vi "Export dat - tag.vi"(8 "Error In":errorcluster, 9 "Workspace":path, 10 "Index":T1 {"IV"."IV properties"."Settling" min=0.0 max=65535.0; "CV"."CV properties"."V range" items=["10mV"=0.01, "100mV"=0.1, "1V"=1.0, "10V"=10.0]; "CV"."CV properties"."I range" items=["100nA"=-7.0, "1µA"=-6.0, "10µA"=-5.0, "100µA"=-4.0, "1mA"=-3.0, "10mA"=-2.0]; "LDLTS"."LDLTS properties"."V range" items=["10mV"=0.01, "100mV"=0.1, "1V"=1.0, "10V"=10.0]; "LDLTS"."LDLTS properties"."I range" items=["100nA"=-7.0, "1µA"=-6.0, "10µA"=-5.0, "100µA"=-4.0, "1mA"=-3.0, "10mA"=-2.0]; "Conv DLTS"."DLTS properties"."V range" items=["10mV"=0.01, "100mV"=0.1, "1V"=1.0, "10V"=10.0]; "Conv DLTS"."DLTS properties"."I range" items=["10mV"=0.01, "100mV"=0.1, "1V"=1.0, "10V"=10.0]}, 11 "Measurement tag":string) -> (0 "Error Out":errorcluster)   [LabVIEW 2019]
doc: "Handles export of measurement (identified by a tag) to a .dat file, displays a GUI window"
uses:
  Type defs/Session internal index Type Def.ctl
  Type defs/IV measurement Type Def.ctl
  Type defs/IV properties Type Def.ctl
  Type defs/CV measurement Type Def.ctl
  Type defs/CV properties Type Def.ctl
  Type defs/LDLTS measurement Type Def.ctl
  Type defs/LDLTS properties Type Def.ctl
  Type defs/cDLTS measurement Type Def.ctl
  Type defs/DLTS properties Type Def.ctl
  <vilib>/Utility/sysdir.llb/System Directory Type.ctl
  <vilib>/Utility/file.llb/Write Delimited Spreadsheet (string).vi
  <vilib>/Utility/file.llb/Write Delimited Spreadsheet (DBL).vi
panel:
  out "String":string
  in  "Path":path caption="Export file as:"
  in  "Export":bool
  in  "Cancel":bool
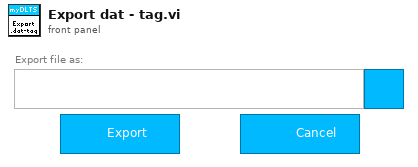
[diagram p1: front panel]
types:
  T1 = typedef "Session internal index Type Def.ctl" = cluster{"IV":T2[], "CV":T4[], "LDLTS":T6[], "Conv DLTS":T8[]}
  T2 = typedef "IV measurement Type Def.ctl" = cluster{"Name":string, "Comment":string, "Time":timestamp, "Folder":path, "IV properties":T3, "GUID":string}
  T3 = typedef "IV properties Type Def.ctl" = cluster{"T":dbl[unit], "Vstart":dbl[unit], "Vstop":dbl[unit], "Vpoints":dbl, "Settling":dbl[unit], "I limit":dbl[unit], "Log mapping":bool, "Averaging":dbl}
  T4 = typedef "CV measurement Type Def.ctl" = cluster{"Name":string, "Comment":string, "Time":timestamp, "Folder":path, "CV properties":T5, "GUID":string}
  T5 = typedef "CV properties Type Def.ctl" = cluster{"T":dbl[unit], "Vstart":dbl[unit], "Vstop":dbl[unit], "Vpoints":dbl, "Precision":enum16{"Low (Fast)", "Normal", "High (Slow)"}, "Test signal":dbl[unit], "Auto I range":bool, "Test frequency":dbl[unit], "I range":dbl, "V range":dbl[unit], "Log mapping":bool, "Rel perm":dbl, "Area":dbl[unit]}
  T6 = typedef "LDLTS measurement Type Def.ctl" = cluster{"Name":string, "Comment":string, "Time":timestamp, "Folder":path, "LDLTS properties":T7, "GUID":string}
  T7 = typedef "LDLTS properties Type Def.ctl" = cluster{"T":dbl[unit], "Test signal":dbl[unit], "Test frequency":dbl[unit], "Bandwidth":dbl[unit], "Averaging":dbl, "Vbias":dbl[unit], "Vpulse":dbl[unit], "pulse length":dbl[unit], "Pulse 2":bool, "Vpulse 2":dbl[unit], "pulse length 2":dbl[unit], "I range":dbl, "V range":dbl[unit], "Sampling rate":dbl[unit], "Acq. delay":dbl[unit], "Sampling time":dbl[unit]}
  T8 = typedef "cDLTS measurement Type Def.ctl" = cluster{"Name":string, "Comment":string, "Time":timestamp, "Folder":path, "DLTS properties":T9, "GUID":string}
  T9 = typedef "DLTS properties Type Def.ctl" = cluster{"Tstart":dbl[unit], "Instant start":bool, "Tstop":dbl[unit], "T rate":dbl[unit], "Test signal":dbl[unit], "Test frequency":dbl[unit], "Bandwidth":dbl[unit], "Averaging":dbl, "Vbias":dbl[unit], "Vpulse":dbl[unit], "pulse length":dbl[unit], "Pulse 2":bool, "Vpulse 2":dbl[unit], "pulse length 2":dbl[unit], "I range":dbl, "V range":dbl[unit], "Emission rate":dbl[unit][], "Sampling rate":dbl[unit], "Acq. delay":dbl[unit]}
  T10 = enum32{"existing file", "new file", "new or existing file", "existing dir", "new dir", "new or existing dir", "existing file (use LLBs)", "new file (use LLBs)", "new or existing file (use LLBs)", "new or existing file or directory (use LLBs)", "existing dir (use LLBs)", "new dir (use LLBs)", "new or existing dir (use LLBs)", "existing file or dir", "new file or dir", "new or existing file or dir", "existing file or dir (use LLBs)", "new file or dir (use LLBs)"}
  T11 = typedef "System Directory Type.ctl" = i32
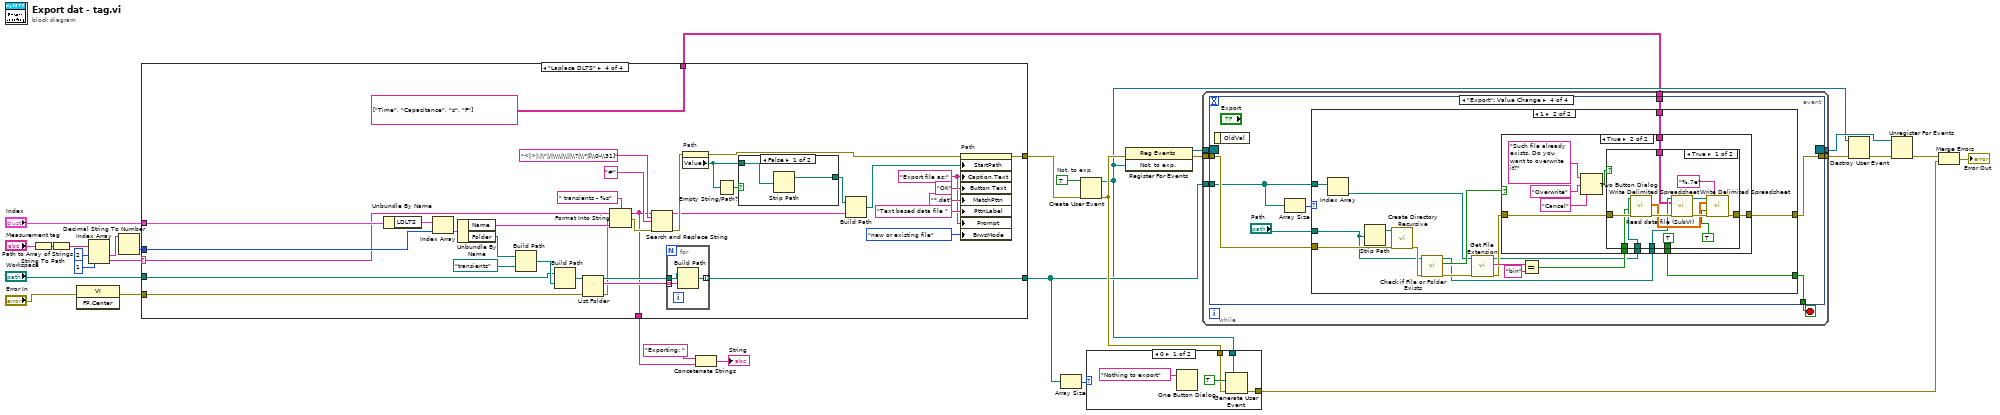
[diagram p0: block diagram]
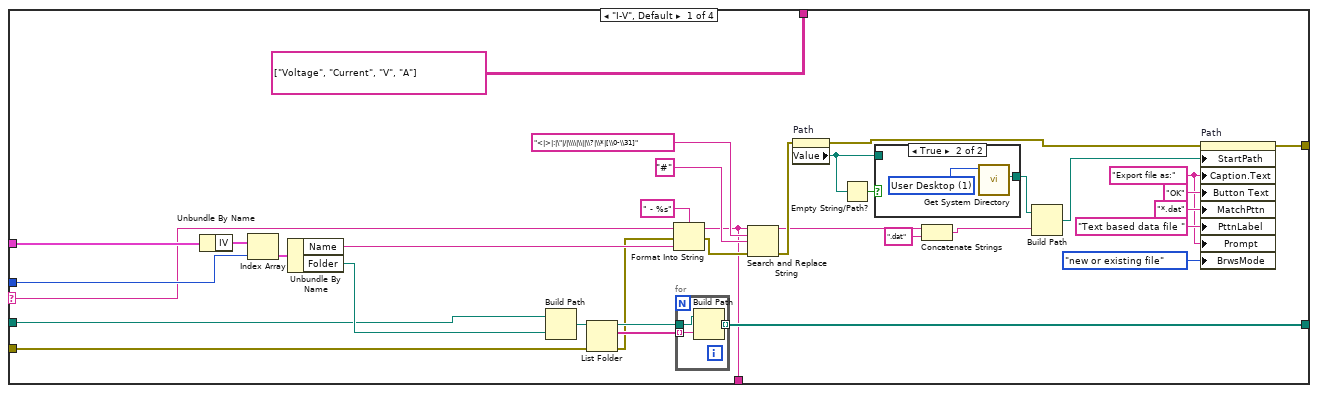
[diagram p3: hidden frame]
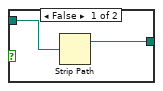
[diagram p4: hidden frame]
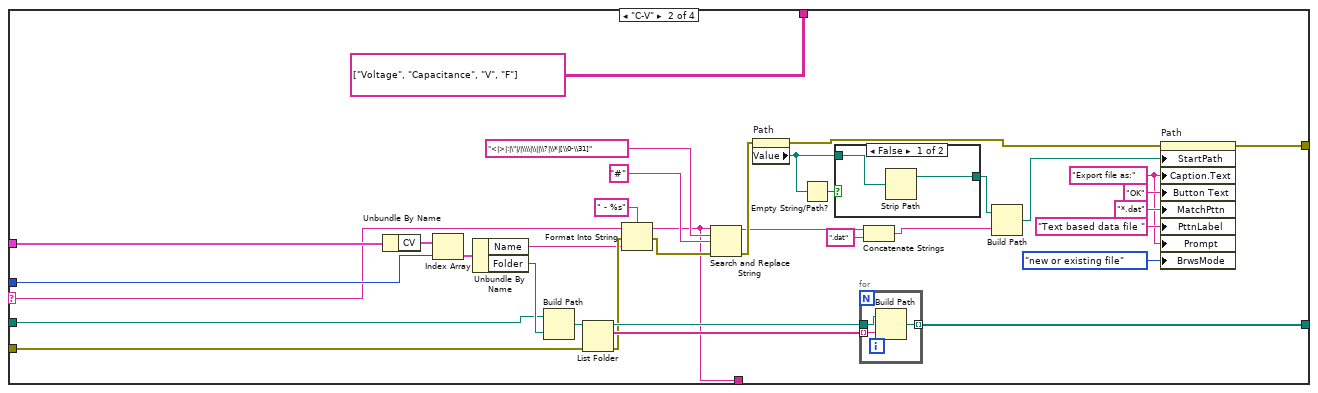
[diagram p5: hidden frame]
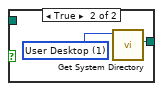
[diagram p6: hidden frame]
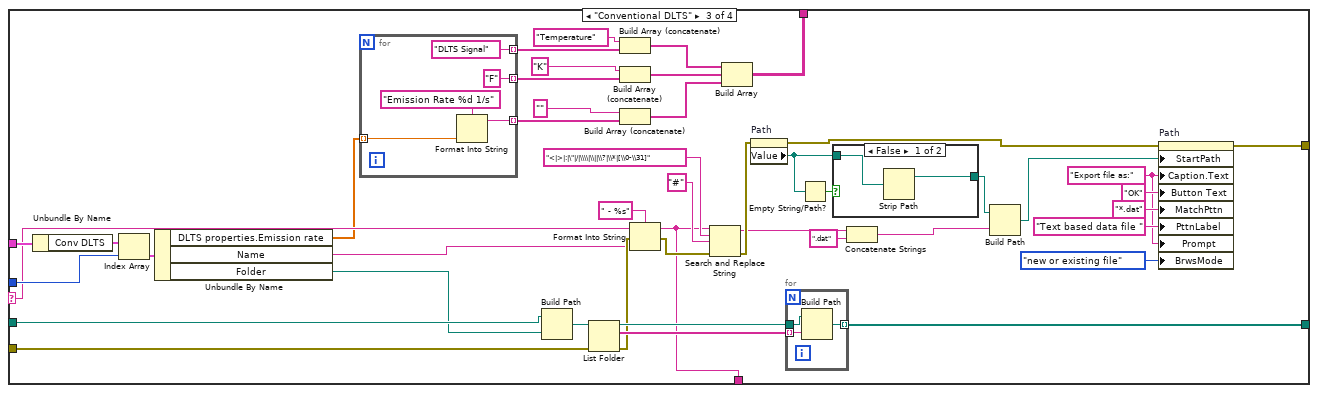
[diagram p7: hidden frame]
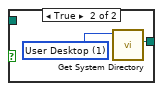
[diagram p8: hidden frame]
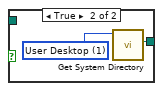
[diagram p9: hidden frame]
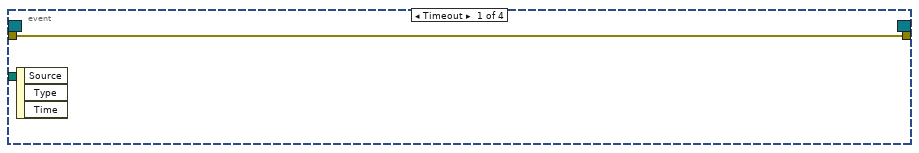
[diagram p10: hidden frame]
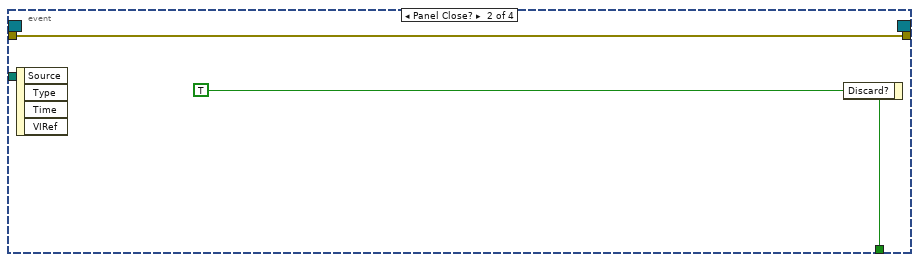
[diagram p11: hidden frame]
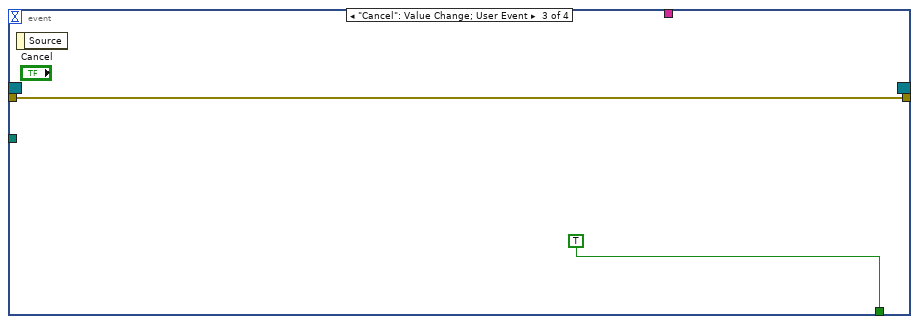
[diagram p12: hidden frame]
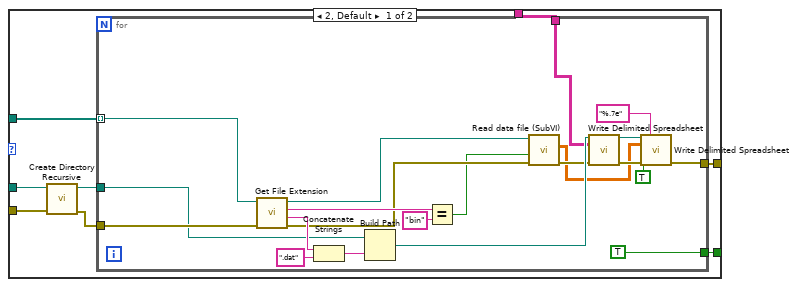
[diagram p13: hidden frame]
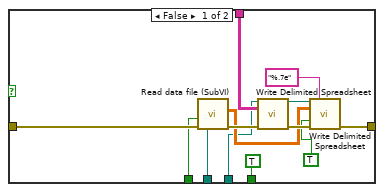
[diagram p14: hidden frame]
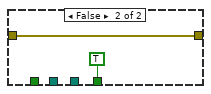
[diagram p15: hidden frame]
diagram:
  w19 = TRUE  # Not. to exp.
  n1 = String To Path(string="Measurement tag") -> (path=w30:path)
  n2 = Path to Array of Strings(0:w30) -> (2:w29:string[])  [unwired: 1 out]
  n3 = invoke class="VI" method="FP.Center"(error in="Error In") -> (error out=w2:errorcluster)  [unwired: 2 in, 2 out]
  n4 = Index Array(array=w29, index #1=2 ("index"), index #2=1 ("index")) -> (element #1=w24:string, element #2=w25:string)
  n5 = Decimal String To Number(string=w24) -> (number=w22:i32)  [unwired: 2 in, 1 out]
  n6 = case shown="\"Laplace DLTS\"" w25 {
    selector: w25 -> [w59 w101 w153 w200]
    tunnel: "Index" -> [w65 w107 w159 w206]
    tunnel: w22 -> [w63 w105 w157 w204]
    tunnel: [w51 w93 w146 w193] -> w14
    tunnel: w2 -> [w49 w91 w144 w191]
    tunnel: [w48 w90 w143 w190] -> w16
    tunnel: "Workspace" -> [w40 w82 w135 w180]
    tunnel: [w36 w75 w131 w173] -> w6
    tunnel: [string[][] [["Voltage", "Current"], ["V", "A"]] string[][] [["Voltage", "Capacitance"], ["V", "F"]] w115 string[][] [["Time", "Capacitance"], ["s", "F"]]] -> w1
    frame "I-V", Default {
      w44 = "Export file as:"
      n7 = Unbundle By Name(w65) -> ("IV"=w64:T2[])
      n8 = Index Array(array=w64, index=w63) -> (element=w62:T2)
      n9 = Unbundle By Name(w62) -> ("Name"=w38:string, "Folder"=w52:path)
      n10 = Build Path(base path=w40, name or relative path=w52) -> (appended path=w42:path)
      n11 = List Folder(path=w42, error in=w49) -> (path out=w41:path, filenames=w50:string[], error out=w32:errorcluster)  [unwired: 2 in, 1 out]
      n12 = Format Into String(format string=" - %s", initial string=w59, error in=w32, w38) -> (resulting string=w36:string, error out=w37:errorcluster)
      n13 = for {
        tunnel: w41 -> [w68]
        tunnel: [w67] -> w51 mode=indexing
        tunnel: w50 -> [w66] mode=indexing
        n14 = Build Path(base path=w68, name or relative path=w66) -> (appended path=w67:path)
      }
      n15 = Search and Replace String(input string=w36, search string="<|>|:|\"|/|\\\\|\\||\\?|\\*|[\\0-\\31]", replace string="#" ("replace string (\"\")"), error in=w37) -> (result string=w35:string, error out=w39:errorcluster)  [unwired: 4 in, 2 out]
      n16 = property on="Path" class="Path"(error in=w39) -> (error out=w53:errorcluster, "Value"=w60:path)  [unwired: 1 in, 1 out]
      n17 = Empty String/Path?(string/path=w60) -> (empty?=w61:bool)
      n18 = case shown="True" w61 {
        tunnel: w60 -> [w70 _]
        tunnel: [w69 w71] -> w55
        frame False {
          n19 = Strip Path(path=w70) -> (stripped path=w69:path)  [unwired: 1 out]
        }
        frame True {
          w72 = T11 1 items=["User Home"=0, "User Desktop"=1, "User Documents"=2, "User Application Data"=3, "User Preferences"=4, "User Temporary"=5, "Public Documents"=6, "Public Application Data"=7, "Public Preferences"=8, "Public Cache"=13, "System Core Libraries"=9, "System Installed Libraries"=10, "Application Files"=11, "Boot Volume Root"=12] ("system directory type")
          n20 = call <vilib>:"Get System Directory.vi"("system directory type"=w72) -> ("system directory"=w71:path)  [unwired: 10 in]
        }
      }
      n21 = Concatenate Strings(w35, ".dat" ("string")) -> (w34:string)
      n22 = Build Path(base path=w55, name or relative path=w34) -> (appended path=w54:path)
      n23 = property on="Path" class="Path"(error in=w53, "StartPath"=w54, "Caption.Text"=w44, "Button Text"="OK", "MatchPttn"="*.dat", "PttnLabel"="Text based data file ", "Prompt"=w44, "BrwsMode"=T10."new or existing file" ("Browse Options:Selection Mode")) -> (error out=w48:errorcluster)  [unwired: 1 in, 1 out]
    }
    frame "C-V" {
      w86 = "Export file as:"
      n24 = Unbundle By Name(w107) -> ("CV"=w106:T4[])
      n25 = Index Array(array=w106, index=w105) -> (element=w104:T4)
      n26 = Unbundle By Name(w104) -> ("Name"=w76:string, "Folder"=w94:path)
      n27 = Build Path(base path=w82, name or relative path=w94) -> (appended path=w84:path)
      n28 = List Folder(path=w84, error in=w91) -> (path out=w83:path, filenames=w92:string[], error out=w78:errorcluster)  [unwired: 2 in, 1 out]
      n29 = Format Into String(format string=" - %s", initial string=w101, error in=w78, w76) -> (resulting string=w75:string, error out=w77:errorcluster)
      n30 = Search and Replace String(input string=w75, search string="<|>|:|\"|/|\\\\|\\||\\?|\\*|[\\0-\\31]", replace string="#" ("replace string (\"\")"), error in=w77) -> (result string=w74:string, error out=w79:errorcluster)  [unwired: 4 in, 2 out]
      n31 = property on="Path" class="Path"(error in=w79) -> (error out=w95:errorcluster, "Value"=w102:path)  [unwired: 1 in, 1 out]
      n32 = Empty String/Path?(string/path=w102) -> (empty?=w103:bool)
      n33 = case shown="False" w103 {
        tunnel: w102 -> [w112 _]
        tunnel: [w111 w113] -> w97
        frame False {
          n34 = Strip Path(path=w112) -> (stripped path=w111:path)  [unwired: 1 out]
        }
        frame True {
          w114 = T11 1 items=["User Home"=0, "User Desktop"=1, "User Documents"=2, "User Application Data"=3, "User Preferences"=4, "User Temporary"=5, "Public Documents"=6, "Public Application Data"=7, "Public Preferences"=8, "Public Cache"=13, "System Core Libraries"=9, "System Installed Libraries"=10, "Application Files"=11, "Boot Volume Root"=12] ("system directory type")
          n35 = call <vilib>:"Get System Directory.vi"("system directory type"=w114) -> ("system directory"=w113:path)  [unwired: 10 in]
        }
      }
      n36 = for {
        tunnel: w83 -> [w110]
        tunnel: [w109] -> w93 mode=indexing
        tunnel: w92 -> [w108] mode=indexing
        n37 = Build Path(base path=w110, name or relative path=w108) -> (appended path=w109:path)
      }
      n38 = Concatenate Strings(w74, ".dat" ("string")) -> (w80:string)
      n39 = Build Path(base path=w97, name or relative path=w80) -> (appended path=w96:path)
      n40 = property on="Path" class="Path"(error in=w95, "StartPath"=w96, "Caption.Text"=w86, "Button Text"="OK", "MatchPttn"="*.dat", "PttnLabel"="Text based data file ", "Prompt"=w86, "BrwsMode"=T10."new or existing file" ("Browse Options:Selection Mode")) -> (error out=w90:errorcluster)  [unwired: 1 in, 1 out]
    }
    frame "Conventional DLTS" {
      w139 = "Export file as:"
      n41 = Unbundle By Name(w159) -> ("Conv DLTS"=w158:T8[])
      n42 = Index Array(array=w158, index=w157) -> (element=w156:T8)
      n43 = Unbundle By Name(w156) -> ("DLTS properties.Emission rate"=w116:dbl[unit][], "Name"=w127:string, "Folder"=w117:path)
      n44 = for {
        tunnel: w116 -> [w164] mode=indexing
        tunnel: [w162] -> w123 mode=indexing
        tunnel: ["DLTS Signal"] -> w121 mode=indexing
        tunnel: ["F"] -> w122 mode=indexing
        n45 = Format Into String(format string="Emission Rate %d 1/s", w164) -> (resulting string=w162:string)  [unwired: 2 in, 1 out]
      }
      n46 = Build Path(base path=w135, name or relative path=w117) -> (appended path=w136:path)
      n47 = List Folder(path=w136, error in=w144) -> (path out=w137:path, filenames=w145:string[], error out=w134:errorcluster)  [unwired: 2 in, 1 out]
      n48 = Build Array (concatenate)("Temperature", w121) -> (w118:string[])
      n49 = Build Array (concatenate)("K", w122) -> (w119:string[])
      n50 = Build Array (concatenate)("", w123) -> (w120:string[])
      n51 = Format Into String(format string=" - %s", initial string=w153, error in=w134, w127) -> (resulting string=w131:string, error out=w133:errorcluster)
      n52 = Search and Replace String(input string=w131, search string="<|>|:|\"|/|\\\\|\\||\\?|\\*|[\\0-\\31]", replace string="#" ("replace string (\"\")"), error in=w133) -> (result string=w128:string, error out=w132:errorcluster)  [unwired: 4 in, 2 out]
      n53 = Build Array(w118, w119, w120) -> (w115:string[][])
      n54 = property on="Path" class="Path"(error in=w132) -> (error out=w147:errorcluster, "Value"=w154:path)  [unwired: 1 in, 1 out]
      n55 = for {
        tunnel: w137 -> [w167]
        tunnel: [w166] -> w146 mode=indexing
        tunnel: w145 -> [w165] mode=indexing
        n56 = Build Path(base path=w167, name or relative path=w165) -> (appended path=w166:path)
      }
      n57 = Empty String/Path?(string/path=w154) -> (empty?=w155:bool)
      n58 = case shown="False" w155 {
        tunnel: w154 -> [w169 _]
        tunnel: [w168 w170] -> w149
        frame False {
          n59 = Strip Path(path=w169) -> (stripped path=w168:path)  [unwired: 1 out]
        }
        frame True {
          w171 = T11 1 items=["User Home"=0, "User Desktop"=1, "User Documents"=2, "User Application Data"=3, "User Preferences"=4, "User Temporary"=5, "Public Documents"=6, "Public Application Data"=7, "Public Preferences"=8, "Public Cache"=13, "System Core Libraries"=9, "System Installed Libraries"=10, "Application Files"=11, "Boot Volume Root"=12] ("system directory type")
          n60 = call <vilib>:"Get System Directory.vi"("system directory type"=w171) -> ("system directory"=w170:path)  [unwired: 10 in]
        }
      }
      n61 = Concatenate Strings(w128, ".dat" ("string")) -> (w129:string)
      n62 = Build Path(base path=w149, name or relative path=w129) -> (appended path=w148:path)
      n63 = property on="Path" class="Path"(error in=w147, "StartPath"=w148, "Caption.Text"=w139, "Button Text"="OK", "MatchPttn"="*.dat", "PttnLabel"="Text based data file ", "Prompt"=w139, "BrwsMode"=T10."new or existing file" ("Browse Options:Selection Mode")) -> (error out=w143:errorcluster)  [unwired: 1 in, 1 out]
    }
    frame "Laplace DLTS" {
      w186 = "Export file as:"
      n64 = Unbundle By Name(w206) -> ("LDLTS"=w205:T6[])
      n65 = Index Array(array=w205, index=w204) -> (element=w203:T6)
      n66 = Unbundle By Name(w203) -> ("Name"=w178:string, "Folder"=w183:path)
      n67 = Build Path(base path=w183, name or relative path=path "transients") -> (appended path=w181:path)
      n68 = Build Path(base path=w180, name or relative path=w181) -> (appended path=w184:path)
      n69 = List Folder(path=w184, error in=w191) -> (path out=w179:path, filenames=w192:string[], error out=w177:errorcluster)  [unwired: 2 in, 1 out]
      n70 = Format Into String(format string=" transients - %s", initial string=w200, error in=w177, w178) -> (resulting string=w173:string, error out=w176:errorcluster)
      n71 = Search and Replace String(input string=w173, search string="<|>|:|\"|/|\\\\|\\||\\?|\\*|[\\0-\\31]", replace string="#" ("replace string (\"\")"), error in=w176) -> (result string=w174:string, error out=w175:errorcluster)  [unwired: 4 in, 2 out]
      n72 = for {
        tunnel: w179 -> [w209]
        tunnel: [w208] -> w193 mode=indexing
        tunnel: w192 -> [w207] mode=indexing
        n73 = Build Path(base path=w209, name or relative path=w207) -> (appended path=w208:path)
      }
      n74 = property on="Path" class="Path"(error in=w175) -> (error out=w194:errorcluster, "Value"=w201:path)  [unwired: 1 in, 1 out]
      n75 = Empty String/Path?(string/path=w201) -> (empty?=w202:bool)
      n76 = case shown="False" w202 {
        tunnel: w201 -> [w211 _]
        tunnel: [w210 w212] -> w196
        frame False {
          n77 = Strip Path(path=w211) -> (stripped path=w210:path)  [unwired: 1 out]
        }
        frame True {
          w213 = T11 1 items=["User Home"=0, "User Desktop"=1, "User Documents"=2, "User Application Data"=3, "User Preferences"=4, "User Temporary"=5, "Public Documents"=6, "Public Application Data"=7, "Public Preferences"=8, "Public Cache"=13, "System Core Libraries"=9, "System Installed Libraries"=10, "Application Files"=11, "Boot Volume Root"=12] ("system directory type")
          n78 = call <vilib>:"Get System Directory.vi"("system directory type"=w213) -> ("system directory"=w212:path)  [unwired: 10 in]
        }
      }
      n79 = Build Path(base path=w196, name or relative path=w174) -> (appended path=w195:path)
      n80 = property on="Path" class="Path"(error in=w194, "StartPath"=w195, "Caption.Text"=w186, "Button Text"="OK", "MatchPttn"="*.dat", "PttnLabel"="Text based data file ", "Prompt"=w186, "BrwsMode"=T10."new or existing file" ("Browse Options:Selection Mode")) -> (error out=w190:errorcluster)  [unwired: 1 in, 1 out]
    }
  }
  n81 = Concatenate Strings("Exporting: " ("string"), w6) -> (→"String":string)
  n82 = Array Size(array=w14) -> (size(s)=w20:i32)
  n83 = Create User Event(user event datatype=w19, error in=w16) -> (user event=w10:refnum<user-event>, error out=w15:errorcluster)
  n84 = case shown="0" w20 {
    tunnel: w10 -> [w217 _]
    tunnel: w15 -> [w215 w219]
    tunnel: [w214 w219] -> w7
    frame 0 {
      n85 = One Button Dialog(message="Nothing to export") -> ()  [unwired: 1 in, 1 out]
      n86 = Generate User Event(user event=w217, event data cluster=TRUE ("event data"), error in=w215) -> (error out=w214:errorcluster)  [unwired: 1 in, 1 out]
    }
    frame 1, Default {
    }
  }
  n87 = register-events(error in=w15, w10) -> (reference out=w17:refnum<event-registration>, error out=w18:errorcluster)  [unwired: 1 in]
  n88 = while {
    tunnel: w18 -> [w226]
    tunnel: [w225] -> w13
    tunnel: w14 -> [w223]
    tunnel: w17 -> [w222]
    tunnel: [w221] -> w11
    tunnel: w1 -> [w220]
    stop <- w224 stop-if-true
    n89 = event shown="[3] \"Export\": Value Change" {
      selector: w222 -> [_ _ _ _]
      dyn-events: [_ _ _ _] -> w221
      timeout: _ -> [_ _ _ _]
      tunnel: w226 -> [w227 w228 w230 w236]
      tunnel: [w227 w228 w230 w238] -> w225
      tunnel: [_ w229 TRUE ("Discard?") w237] -> w224
      tunnel: w223 -> [_ _ _ w233]
      tunnel: w220 -> [_ _ _ w232]
      event Timeout {
        n90 = event-data() -> ()  [unwired: 1 in, 3 out]
      }
      event Panel Close? {
        w229 = TRUE ("Discard?")
        n91 = event-data() -> ()  [unwired: 1 in, 4 out]
        n92 = event-data("Discard?"=w229) -> ()  [unwired: 1 in, 1 out]
      }
      event "Cancel": Value Change; User Event {
        n93 = event-data() -> ()  [unwired: 1 in, 1 out]
      }
      event "Export": Value Change {
        n94 = event-data() -> ()  [unwired: 1 in, 1 out]
        n95 = Array Size(array=w233) -> (size(s)=w234:i32)
        n96 = case shown="1" w234 {
          tunnel: [w246 w276] -> w237
          tunnel: w236 -> [w243 w273]
          tunnel: w233 -> [w245 w272]
          tunnel: "Path" -> [w242 w269]
          tunnel: [w244 w270] -> w238
          tunnel: w232 -> [w239 w268]
          frame 2, Default {
            n97 = call <vilib>:"Create Directory Recursive.vi"("error in (no error)"=w243, "directory"=w242) -> ("error out"=w241:errorcluster, "directory copy"=w240:path)  [unwired: 3 in, 1 out]
            n98 = for {
              tunnel: [TRUE] -> w246
              tunnel: w245 -> [w264] mode=indexing
              tunnel: [w250] -> w244
              tunnel: w241 -> [w260]
              tunnel: w240 -> [w259]
              tunnel: w239 -> [w247]
              n99 = call <vilib>:"Get File Extension.vi"("error in (no error)"=w260, "file"=w264) -> ("error out"=w254:errorcluster, "filename without extension"=w262:string, "lowercase file extension"=w267:string, "dup file"=w255:path)  [unwired: 5 in, 1 out]
              n100 = Concatenate Strings(w262, ".dat" ("string")) -> (w263:string)
              n101 = Build Path(base path=w259, name or relative path=w263) -> (appended path=w252:path)
              n102 = Equal?(x=w267, y="bin") -> (x = y?=w253:bool)
              n103 = call "Read data file (SubVI).vi"("error in"=w254, "Binary"=w253, "file path in"=w255) -> ("error out"=w249:errorcluster, "2D data"=w248:dbl[][])  [unwired: 6 in, 1 out]
              n104 = call-poly <vilib>:"Write Delimited Spreadsheet.vi"("file path (dialog if empty)"=w252, "2D data"=w247, "error in (no error)"=w249) -> ("new file path (Not A Path if cancelled)"=w251:path, "error out"=w257:errorcluster)  [unwired: 11 in]
              n105 = call-poly <vilib>:"Write Delimited Spreadsheet.vi"("file path (dialog if empty)"=w251, "format (%.3f)"="%.7e", "2D data"=w248, "append to file? (new file:F)"=TRUE, "error in (no error)"=w257) -> ("error out"=w250:errorcluster)  [unwired: 9 in, 1 out]
            }
          }
          frame 1 {
            n106 = Index Array(array=w272) -> (element=w271:path)  [unwired: 1 in]
            n107 = Strip Path(path=w269) -> (stripped path=w275:path)  [unwired: 1 out]
            n108 = call <vilib>:"Create Directory Recursive.vi"("error in (no error)"=w273, "directory"=w275) -> ("error out"=w274:errorcluster)  [unwired: 3 in, 2 out]
            n109 = call <vilib>:"Check if File or Folder Exists.vi"("error in (no error)"=w274, "path"=w269) -> ("error out"=w279:errorcluster, "file or folder exists?"=w284:bool, "dup path"=w277:path)  [unwired: 7 in]
            n110 = call <vilib>:"Get File Extension.vi"("error in (no error)"=w279, "file"=w271) -> ("error out"=w280:errorcluster, "lowercase file extension"=w283:string, "dup file"=w278:path)  [unwired: 5 in, 2 out]
            n111 = Equal?(x=w283, y="bin") -> (x = y?=w282:bool)
            n112 = case shown="True" w284 {
              tunnel: [w290 w308] -> w270
              tunnel: [TRUE w307] -> w276
              tunnel: w280 -> [w288 w302]
              tunnel: w277 -> [w285 w301]
              tunnel: w278 -> [w286 w300]
              tunnel: w282 -> [w287 w299]
              tunnel: w268 -> [w289 w298]
              frame False {
                n113 = call "Read data file (SubVI).vi"("error in"=w288, "Binary"=w287, "file path in"=w286) -> ("error out"=w293:errorcluster, "2D data"=w292:dbl[][])  [unwired: 6 in, 1 out]
                n114 = call-poly <vilib>:"Write Delimited Spreadsheet.vi"("file path (dialog if empty)"=w285, "2D data"=w289, "error in (no error)"=w293) -> ("new file path (Not A Path if cancelled)"=w294:path, "error out"=w296:errorcluster)  [unwired: 11 in]
                n115 = call-poly <vilib>:"Write Delimited Spreadsheet.vi"("file path (dialog if empty)"=w294, "format (%.3f)"="%.7e", "2D data"=w292, "append to file? (new file:F)"=TRUE, "error in (no error)"=w296) -> ("error out"=w290:errorcluster)  [unwired: 9 in, 1 out]
              }
              frame True {
                n116 = Two Button Dialog(message="Such file already exists. Do you want to overwrite it?", 1:"Cancel" ("F button name (\"Cancel\")"), 2:"Overwrite" ("T button name (\"OK\")")) -> (T button?=w303:bool)
                n117 = case shown="True" w303 {
                  tunnel: [w314 w322] -> w308
                  tunnel: [TRUE TRUE] -> w307
                  tunnel: w302 -> [w315 w322]
                  tunnel: w301 -> [w313 _]
                  tunnel: w300 -> [w312 _]
                  tunnel: w299 -> [w311 _]
                  tunnel: w298 -> [w309 _]
                  frame True {
                    n118 = call "Read data file (SubVI).vi"("error in"=w315, "Binary"=w311, "file path in"=w312) -> ("error out"=w317:errorcluster, "2D data"=w316:dbl[][])  [unwired: 6 in, 1 out]
                    n119 = call-poly <vilib>:"Write Delimited Spreadsheet.vi"("file path (dialog if empty)"=w313, "2D data"=w309, "error in (no error)"=w317) -> ("new file path (Not A Path if cancelled)"=w318:path, "error out"=w320:errorcluster)  [unwired: 11 in]
                    n120 = call-poly <vilib>:"Write Delimited Spreadsheet.vi"("file path (dialog if empty)"=w318, "format (%.3f)"="%.7e", "2D data"=w316, "append to file? (new file:F)"=TRUE, "error in (no error)"=w320) -> ("error out"=w314:errorcluster)  [unwired: 9 in, 1 out]
                  }
                  frame False {
                  }
                }
              }
            }
          }
        }
      }
    }
  }
  n121 = Destroy User Event(user event=w10, error in=w13) -> (error out=w12:errorcluster)
  n122 = Unregister For Events(event registration refnum=w11, error in=w12) -> (error out=w9:errorcluster)
  n123 = Merge Errors(w9, w7) -> (→"Error Out":errorcluster)
